vi "TMCM351_setTozero.vi"(3 "错误输入":errorcluster caption="错误输入（无错误）", 4 "归0到位":bool[](array[boolean]), 5 "com in":refnum<visa-resource-name>) -> (0 "错误输出":errorcluster, 2 "com out":refnum<visa-resource-name>)   [LabVIEW 2018]
uses:
  Device VIs/Verbal.vi
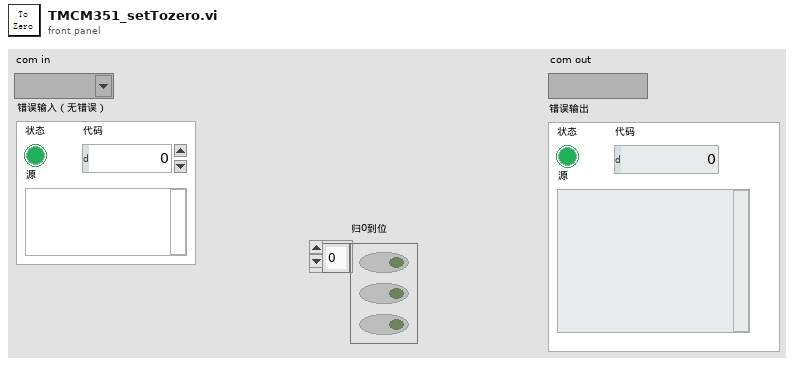
[diagram p1: front panel]
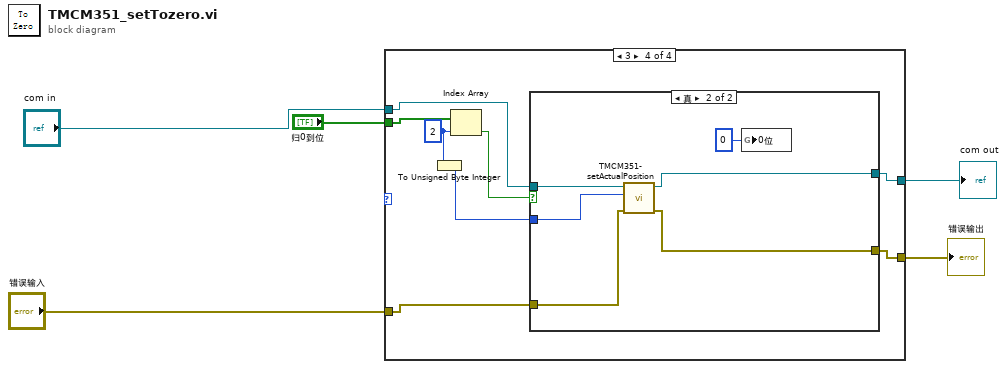
[diagram p0: block diagram]
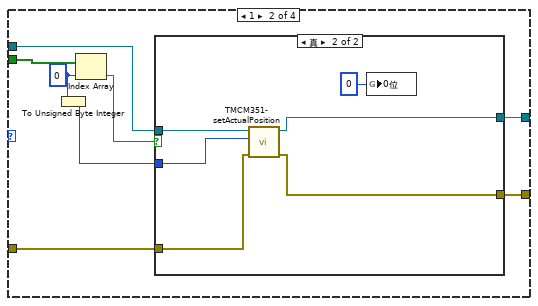
[diagram p3: hidden frame]
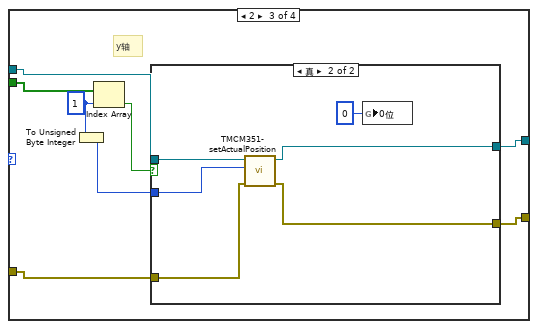
[diagram p5: hidden frame]
diagram:
  n1 = case shown="3" {
    selector: _ -> [_ _ _ _]
    tunnel: "归0到位" -> [_ w15 w29 w45]
    tunnel: "com in" -> [w7 w13 w30 w46]
    tunnel: "错误输入" -> [w6 w12 w28 w44]
    tunnel: [w7 w11 w27 w43] -> w2
    tunnel: [w6 w10 w26 w42] -> w1
    frame 0, Default {
    }
    frame 1 {
      w9 = 0 ("索引")
      n2 = To Unsigned Byte Integer(number=w9) -> (unsigned 8bit integer=w8:u8)
      n3 = Index Array(array=w15, index=w9) -> (element=w14:bool)
      n4 = case shown="真" w14 {
        tunnel: w13 -> [w17 w23]
        tunnel: w12 -> [w16 w22]
        tunnel: [w17 w21] -> w11
        tunnel: [w16 w20] -> w10
        tunnel: w8 -> [_ w18]
        frame False {
        }
        frame True {
          n5 = call "TMCM351- setActualPosition.vi"("错误输入"=w22, "motor"=w18, "com in"=w23) -> ("错误输出"=w20:errorcluster, "com out"=w21:refnum<visa-resource-name>)  [unwired: 3 in]
          n6 = global write "Verbal.vi" "0位"(u8 0 ("0位")) -> ()
        }
      }
    }
    frame 2 {
      w25 = 1 ("索引")
      # "y轴"
      n7 = To Unsigned Byte Integer(number=w25) -> (unsigned 8bit integer=w24:u8)
      n8 = Index Array(array=w29, index=w25) -> (element=w31:bool)
      n9 = case shown="真" w31 {
        tunnel: w30 -> [w33 w39]
        tunnel: w28 -> [w32 w38]
        tunnel: [w33 w37] -> w27
        tunnel: [w32 w36] -> w26
        tunnel: w24 -> [_ w34]
        frame False {
        }
        frame True {
          n10 = call "TMCM351- setActualPosition.vi"("错误输入"=w38, "motor"=w34, "com in"=w39) -> ("错误输出"=w36:errorcluster, "com out"=w37:refnum<visa-resource-name>)  [unwired: 3 in]
          n11 = global write "Verbal.vi" "0位"(u8 0 ("0位")) -> ()
        }
      }
    }
    frame 3 {
      w41 = 2 ("索引")
      n12 = To Unsigned Byte Integer(number=w41) -> (unsigned 8bit integer=w40:u8)
      n13 = Index Array(array=w45, index=w41) -> (element=w47:bool)
      n14 = case shown="真" w47 {
        tunnel: w46 -> [w49 w55]
        tunnel: w44 -> [w48 w54]
        tunnel: [w49 w53] -> w43
        tunnel: [w48 w52] -> w42
        tunnel: w40 -> [_ w50]
        frame False {
        }
        frame True {
          n15 = call "TMCM351- setActualPosition.vi"("错误输入"=w54, "motor"=w50, "com in"=w55) -> ("错误输出"=w52:errorcluster, "com out"=w53:refnum<visa-resource-name>)  [unwired: 3 in]
          n16 = global write "Verbal.vi" "0位"(u8 0 ("0位")) -> ()
        }
      }
    }
  }
  "com out" <- w2
  "错误输出" <- w1
